vi "Wait For Signal Bank To Write.vi"(8 "error in (no error)":errorcluster, 10 "timeout (ms)":i32=5000) -> (0 "error out":errorcluster={"status"=FALSE, "code"=0, "source"="."}, 2 "Time":i32)   [LabVIEW 2020]
uses:
  PXI Globals.vi
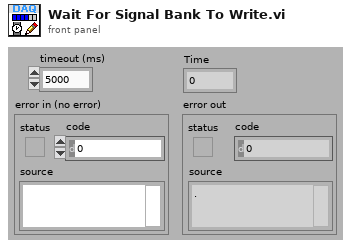
[diagram p1: front panel]
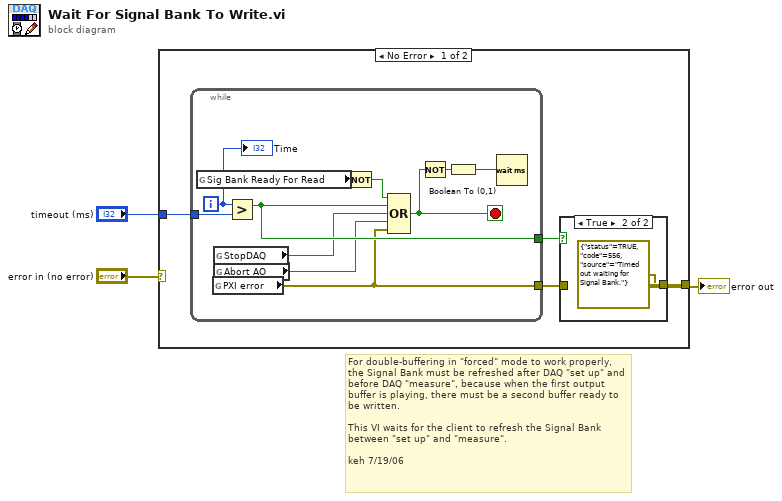
[diagram p0: block diagram]
diagram:
  # "For double-buffering in \"forced\" mode to work properly, the Signal Bank must be refreshed after DAQ \"set up\" and before DAQ \"measure\", because when the first output buffer is playing, there must be a second buffer ready to be written. \n\nThis VI waits for the client to refresh the Signal Bank between \"set up\" and \"measure\".\n\nkeh 7/19/06"
  n1 = case shown="No Error" "error in (no error)" {
    selector: "error in (no error)" -> [_ w21]
    tunnel: [w6 w21] -> w3
    tunnel: "timeout (ms)" -> [w5 _]
    frame No Error {
      n2 = while {
        tunnel: w5 -> [w17]
        tunnel: [w18] -> w7
        tunnel: [w14] -> w4
        i -> [w19]
        stop <- w13 stop-if-true
        n3 = global read "PXI Globals.vi" "Sig Bank Ready For Read"() -> (w20:bool)
        n4 = global read "PXI Globals.vi" "PXI error"() -> (w14:errorcluster)
        n5 = global read "PXI Globals.vi" "StopDAQ"() -> (w16:bool)
        n6 = global read "PXI Globals.vi" "Abort AO"() -> (w10:bool)
        n7 = Greater?(x=w19, y=w17) -> (0:w18:bool)
        n8 = Not(x=w20) -> (.not. x?=w15:bool)
        n9 = Compound Arithmetic op=OR(w15, w18, w16, w10, w14) -> (w13:bool)
        n10 = Not(x=w13) -> (.not. x?=w12:bool)
        n11 = Boolean To (0,1)(Boolean=w12) -> (0, 1=w11:i16)
        n12 = Wait (ms)(milliseconds to wait=w11) -> ()  [unwired: 1 out]
        "Time" <- w19
      }
      n13 = case shown="True" w7 {
        tunnel: [w8 errorcluster {"status"=TRUE, "code"=556, "source"="Timed out waiting for Signal Bank."} ("error out 2")] -> w6
        tunnel: w4 -> [w8 _]
        frame False {
        }
        frame True {
        }
      }
    }
    frame Error {
    }
  }
  "error out" <- w3
